vi "To String Array.vi"(8 "error in (no error)":errorcluster, 11 "Counter Config in":refnum<class "Counter Config.lvclass">) -> (0 "error out":errorcluster, 1 "Step String Array":string[](array[string]), 3 "Counter Config out":refnum<class "Counter Config.lvclass">)   [LabVIEW 2015, in "Counter Config.lvclass"]
uses:
  Counter Config.lvclass
  <vilib>/NI/Tag Bus/tag/tag descriptor.lvclass/tag descriptor.ctl
  <vilib>/NI/Tag Bus Module Framework/channel/TBM channel.lvclass
  classes/Step/Config/Step Config.lvclass
  <vilib>/NI/Tag Bus/tag/tag descriptor.lvclass
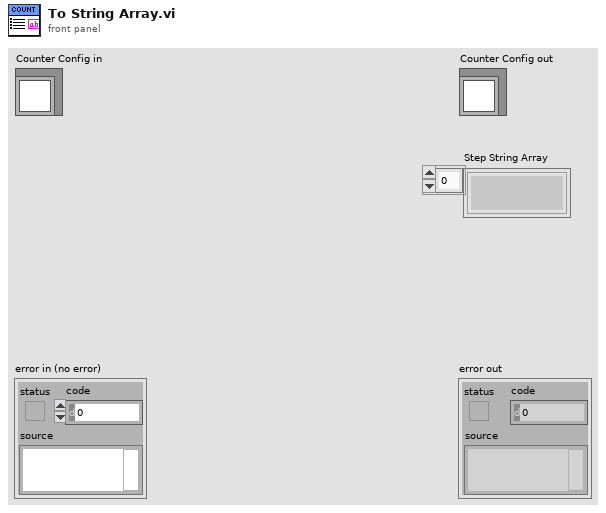
[diagram p1: front panel]
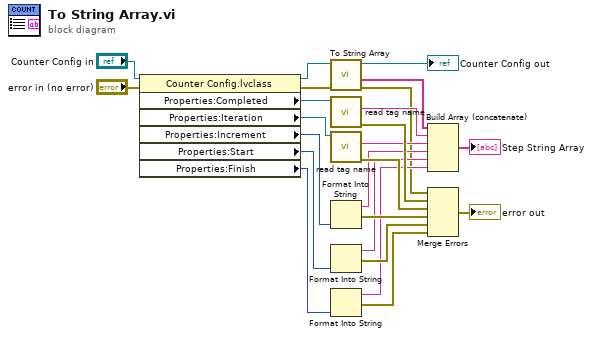
[diagram p0: block diagram]
diagram:
  n1 = property class="Counter Config.lvclass"(reference="Counter Config in", error in="error in (no error)") -> (reference out=w5:refnum<class "Counter Config.lvclass">, error out=w2:errorcluster, "Properties:Completed"=w21:refnum<class "TBM channel.lvclass">, "Properties:Iteration"=w20:refnum<class "TBM channel.lvclass">, "Properties:Increment"=w19:i32, "Properties:Start"=w18:i32, "Properties:Finish"=w17:i32)
  n2 = call-parent "To String Array.vi"("error in (no error)"=w2, "Step Config in"=w5) -> ("error out"=w1:errorcluster, "Step String Array"=w3:string[], "Step Config out"=→"Counter Config out":refnum<class "Counter Config.lvclass">)  [unwired: 7 in]
  n3 = call <vilib>:"read tag name.vi"("system tag in"=w21) -> ("error out"=w16:errorcluster, "name"=w10:string)  [unwired: 8 in, 1 out]
  n4 = call <vilib>:"read tag name.vi"("system tag in"=w20) -> ("error out"=w15:errorcluster, "name"=w9:string)  [unwired: 8 in, 1 out]
  n5 = Format Into String(w19) -> (resulting string=w8:string, error out=w14:errorcluster)  [unwired: 3 in]
  n6 = Format Into String(w18) -> (resulting string=w7:string, error out=w13:errorcluster)  [unwired: 3 in]
  n7 = Format Into String(w17) -> (resulting string=w6:string, error out=w12:errorcluster)  [unwired: 3 in]
  n8 = Build Array (concatenate)(w3, w10, w9, w8, w7, w6) -> (→"Step String Array":string[])
  n9 = Merge Errors(w1, w16, w15, w14, w13, w12) -> (→"error out":errorcluster)
